vi "ConnectionArduino.vi"(8 "error in":errorcluster) -> (0 "error out":errorcluster, 2 "Arduino":bool, 3 "Arduino":refnum<visa-resource-name>)   [LabVIEW 2022 SP3]
uses:
  <vilib>/Instr/_visa.llb/VISA Find Search Mode.ctl
  <vilib>/Instr/_visa.llb/VISA Configure Serial Port (Instr).vi
  <vilib>/regexp/Match Regular Expression.xnode
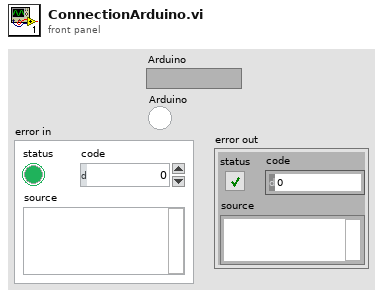
[diagram p1: front panel]
types:
  T1 = typedef "VISA Find Search Mode.ctl" = u32
  T2 = cluster{"VISA resource name":refnum<visa-resource-name>, "error out":errorcluster}
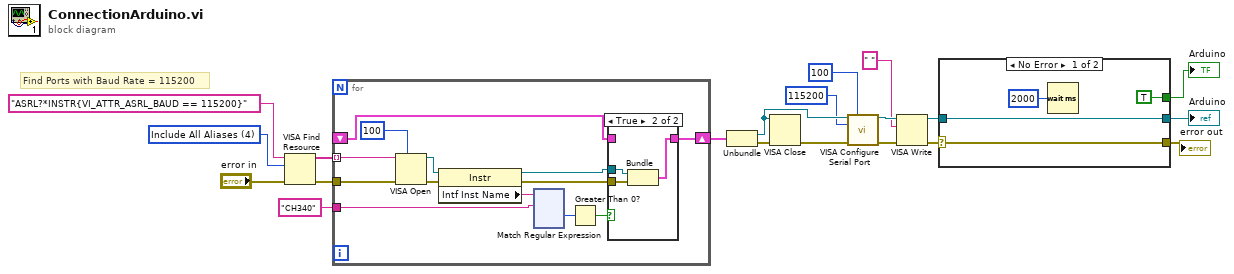
[diagram p0: block diagram]
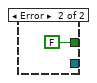
[diagram p2: hidden frame]
diagram:
  w8 = T1 4 items=["Canonical Names Only"=0, "Aliases Only"=2, "Include Matching Aliases"=3, "Include All Aliases"=4] ("Search Mode")
  # "Find Ports with Baud Rate = 115200"
  n1 = VISA Find Resource(8:"error in", 10:w8, 11:"ASRL?*INSTR{VI_ATTR_ASRL_BAUD == 115200}" ("expression (\"?*\")")) -> (0:w17:errorcluster, 3:w20:string[])  [unwired: 1 out]
  n2 = for {
    tunnel: w20 -> [w33] mode=indexing
    tunnel: "CH340" -> [w29]
    shift-right: [w27] -> w19
    shift-left: _ -> [w26]
    tunnel: w17 -> [w25]
    n3 = VISA Open(timeout (0)=u32 100 ("VISA Open timeout (0)"), error in (no error)=w25, VISA resource name=w33) -> (VISA resource name=w32:refnum<visa-resource-name>, error out=w28:errorcluster)  [unwired: 2 in]
    n4 = property class="Instr"(reference=w32, error in=w28) -> (reference out=w24:refnum<visa-resource-name>, error out=w23:errorcluster, "Intf Inst Name"=w22:string)
    n5 = xnode "Match Regular Expression"("input string"=w22, "regular expression"=w29) -> ("offset past match"=w31:i32)  [unwired: 4 in, 4 out]
    n6 = Greater Than 0?(x=w31) -> (x > 0?=w30:bool)
    n7 = case shown="True" w30 {
      tunnel: w24 -> [_ w37]
      tunnel: w23 -> [_ w36]
      tunnel: [w34 w35] -> w27
      tunnel: w26 -> [w34 _]
      frame False {
      }
      frame True {
        n8 = Bundle("VISA resource name"=w37, "error out"=w36) -> (w35:T2)  [unwired: 1 in]
      }
    }
  }
  n9 = Unbundle(w19) -> ("VISA resource name"=w9:refnum<visa-resource-name>, "error out"=w14:errorcluster)
  n10 = VISA Close(VISA resource name=w9, error in (no error)=w14) -> (error out=w13:errorcluster)
  n11 = call-poly "VISA Configure Serial Port"("VISA resource name"=w9, "timeout (10sec)"=u32 100, "baud rate (9600)"=u32 115200, "error in (no error)"=w13) -> ("VISA resource name out"=w12:refnum<visa-resource-name>, "error out"=w11:errorcluster)  [unwired: 10 in]
  n12 = VISA Write(VISA resource name=w12, write buffer=" ", error in (no error)=w11) -> (VISA resource name out=w7:refnum<visa-resource-name>, error out=w6:errorcluster)  [unwired: 1 out]
  n13 = case shown="No Error" w6 {
    selector: w6 -> [w156 _]
    tunnel: [TRUE FALSE] -> w4
    tunnel: w7 -> [w157 _]
    tunnel: [w157 _] -> w5
    tunnel: [w156 _] -> w2
    frame No Error {
      n14 = Wait (ms)(milliseconds to wait=u32 2000) -> ()  [unwired: 1 out]
    }
    frame Error {
    }
  }
  "Arduino" <- w5
  "Arduino" <- w4
  "error out" <- w2
